vi "execute.vi"(2 "error in":errorcluster, 3 "Input":string) -> (0 "error out":errorcluster, 1 "parsed reply":string)   [LabVIEW 2016, in "labssh_thijs.lvlib"]
uses:
  labssh_thijs.lvlib
  Labview SSH driver/state machine.ctl
  Labview SSH driver/store retrieve.ctl
panel:
  out "predetermined prompt without $":string
  out "output_raw":string
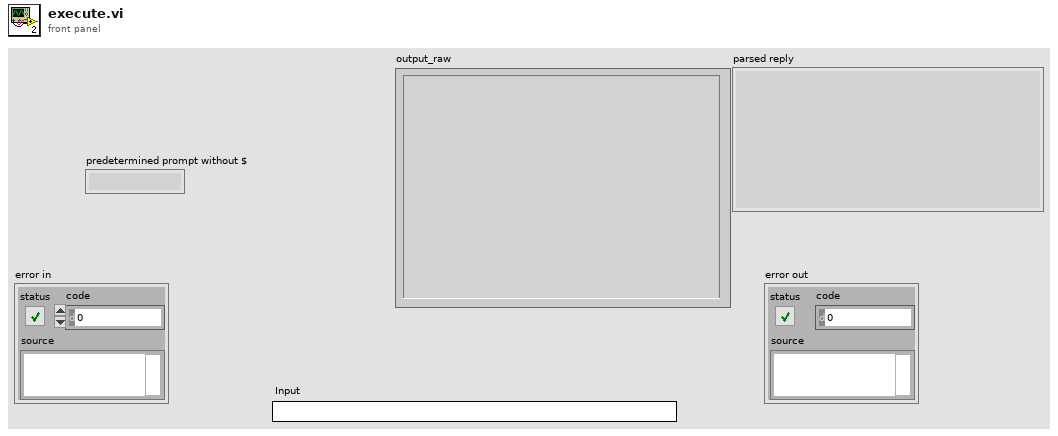
[diagram p1: front panel]
types:
  T1 = typedef "labssh_thijs.lvlib/store retrieve.ctl" = enum16{"store", "retrieve"}
  T2 = typedef "labssh_thijs.lvlib/state machine.ctl" = enum16{"init", "connect", "execute", "close", "exit", "read"}
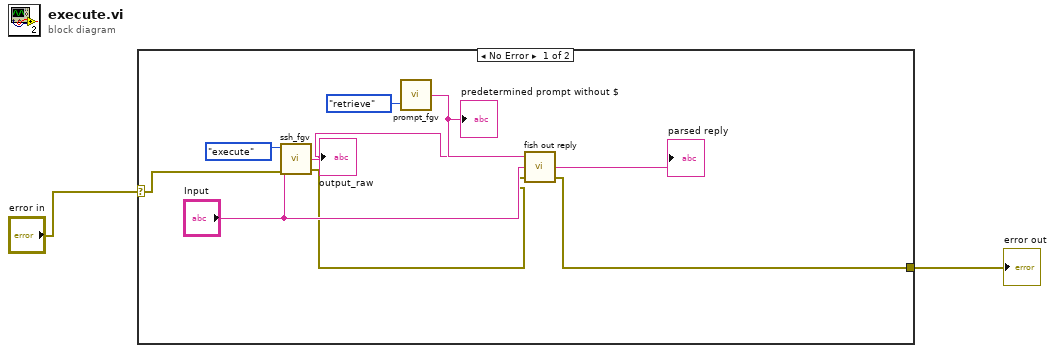
[diagram p0: block diagram]
diagram:
  n1 = case shown="No Error" "error in" {
    selector: "error in" -> [w10 w12]
    tunnel: [w6 w12] -> w1
    frame No Error {
      n2 = call "ssh_fgv.vi"(0:state_machine."execute", "Input"="Input", "error in"=w10) -> ("output_new"=w3:string, "error out"=w7:errorcluster)  [unwired: 4 in]
      "output_raw" <- w3
      n3 = call "prompt_fgv.vi"(1:store_retrieve."retrieve") -> ("String out"=w4:string)  [unwired: 1 in]
      "predetermined prompt without $" <- w4
      n4 = call "fish out reply.vi"("predetermined prompt without $"=w4, "error in"=w7, "original command"="Input", "total output"=w3) -> ("error out"=w6:errorcluster, "final match"=→"parsed reply":string)
    }
    frame Error {
    }
  }
  "error out" <- w1
